vi "SysDef.Compile.vi"(8 "error in (no error)":errorcluster, 11 "Device Reference in":T1 format="%.0x") -> (0 "error out":errorcluster, 1 "Refs":T2(array[cluster]) {"VS Refs" format="%.0x"}, 2 "VS References":T3={"Name"="", "CAN"={"Interface"="", "Baud Rate"=0, "Diagnostic Protocol"=enum."GMLAN", "Transport Protocol"=enum."ISO TP - Normal Mode", "Transmit ID"=0, "Receive ID"=2, "Transmit Extension"=1, "Receive Extension"=255, "Receive UUDT ID"=0, "Enable Stream"=TRUE, "VW TP Channel ID"=1, "Fill Frame"=FALSE, "Fill Byte"=0, "Termination"=FALSE, "LIN Cluster"="", "NAD"=8, "IO Mode"=0, "Max DLC"=0, "FD Baud Rate"=2, "Security"={"Type"=enum."None", "Source DLL Path"=path "", "Target DLL Path"=path "", "Security Level"=0, "Master Key"=""}, "Timeout"=1}, "986x"={"Enable"=FALSE, "RIO Device"="", "Bitfile"=path ""}, "Reads"=[], "Frames Lookup"=variant(enum16{"GMLAN", "KWP-2000", "UDS"} enum."GMLAN"), "Writes"=[], "DPIDs"=[], "DPID Lookup"=variant(u32 0), "DTC"={"Descriptor"={"DTC Byte Length"=1, "Status Byte Length"=1, "Add Data Byte Length"=1, "Byte Order"=enum."Motorola"}, "Value.Code"=[], "Value.String"=[], "Value.J2012String"=[], "Status.Code"=[], "Status.String"=[]}, "Created DTCs"=0, "Polls"=[], "Service Channels Status Lookup"=variant, "Trigger Lookup"=variant} {"Writes"."Signals"."Byte Order" items=["Little Endian", "Big Endian"]; "Writes"."Signals"."Data Type" items=["Signed", "Unsigned", "IEEE Float"]; "CAN"."IO Mode" items=["CAN 2.0", "CAN FD", "CAN FD+BRS"]; "CAN"."Fill Byte" format="%.0x"; "CAN"."VW TP Channel ID" format="%.0x"; "CAN"."Receive UUDT ID" format="%.0x"; "CAN"."Receive Extension" format="%.0x"; "CAN"."Transmit Extension" format="%.0x"; "CAN"."Receive ID" format="%.0x"; "CAN"."Transmit ID" format="%.0x"; "Reads"."Signals"."Byte Order" items=["Little Endian", "Big Endian"]; "Reads"."Signals"."Data Type" items=["Signed", "Unsigned", "IEEE Float"]}, 3 "Device Reference out":T1 format="%.0x")   [LabVIEW 2019, in "Diagnostics Addon System Explorer.lvlib"]
uses:
  Diagnostics Addon System Explorer.lvlib
  <vilib>/NI VeriStand/Custom Device API/Custom Device Item Ref.ctl
  Shared/Types/SysDef.Compile.ctl
  Shared/Types/CAN.ctl
  Shared/Types/CAN.Interface.ctl
  Shared/Types/Protocol.ctl
  Shared/Types/Transport.ctl
  Shared/Types/Security.ctl
  Shared/Types/Security.Type.ctl
  Shared/Types/986x.ctl
  Shared/Types/Frame.Compile.ctl
  Shared/Types/Type.ctl
  Shared/Types/Signal.ctl
  Shared/Types/DPID.ctl
  Shared/Types/DPID.Rate.ctl
  Shared/Types/DTC.Settings.ctl
  Shared/Types/DTC.Descriptor.ctl
  Shared/Types/Poll.Compiled.ctl
  Types/FG.Action.ctl
  Signals.Get.vi
  Type.FG.vi
  ServiceChannels.GetRefs.vi
  SettingChannels.GetRefs.vi
  FileDependency.Create.vi
  Shared/SubVIs/Frame.Get.Size.vi
  Shared/SubVIs/LookupID.Create.vi
  Signal.FG.vi
  Frame.GetSignalRefs.vi
  Shared/SubVIs/Constants.vi
  <vilib>/NI VeriStand/Custom Device Tools/Custom Device Utility Library/NI VeriStand - Search for Item by GUID.vi
  <vilib>/NI VeriStand/Custom Device Tools/Custom Device Utility Library/NI VeriStand - Search for Item by Name.vi
  <vilib>/NI VeriStand/Custom Device API/NI VeriStand - Get Item Children.vi
  <vilib>/NI/NI VeriStand Advanced SysDef API/SysDef API/SysDef.Property.Set.vi
  <vilib>/NI/NI VeriStand Advanced SysDef API/_SubVIs/SysDef.Property.Set.U32.vi
  <vilib>/NI VeriStand/Custom Device API/NI VeriStand - Get Item Property.vi
  <vilib>/NI VeriStand/Custom Device API/Get Item Property (U32).vi
  <vilib>/NI/NI VeriStand Advanced SysDef API/_SubVIs/SysDef.Property.Set.DBL.vi
  <vilib>/NI/NI VeriStand Advanced SysDef API/_SubVIs/SysDef.Property.Set.String.vi
  <vilib>/NI VeriStand/Custom Device API/Get Item Property (Double).vi
  <vilib>/NI VeriStand/Custom Device API/Get Item Property (String).vi
  <vilib>/NI VeriStand/Custom Device API/NI VeriStand - Get Item Description.vi
  <vilib>/NI VeriStand/Custom Device API/NI VeriStand - Get Custom Device Channel Data.vi
  <vilib>/NI VeriStand/Custom Device Tools/Custom Device Utility Library/NI VeriStand - Search for All Items by GUID.vi
  <vilib>/NI/NI VeriStand Advanced SysDef API/_SubVIs/SysDef.Property.Set.I32.vi
  <vilib>/NI/NI VeriStand Advanced SysDef API/_SubVIs/SysDef.Property.Set.DBL.Array.vi
  <vilib>/NI/NI VeriStand Advanced SysDef API/_SubVIs/SysDef.Property.Set.String.Array.vi
  <vilib>/NI VeriStand/Custom Device API/Get Item Property (I32).vi
  <vilib>/NI VeriStand/Custom Device API/Get Item Property (Double Array).vi
  <vilib>/NI VeriStand/Custom Device API/Get Item Property (String Array).vi
  <vilib>/NI VeriStand/Custom Device API/Get Item Property (Variant).vi
  <vilib>/NI VeriStand/Custom Device API/Get Item Property (Boolean).vi
  FileDependency.Get.Target Path.vi
  <vilib>/NI/NI VeriStand Advanced SysDef API/_SubVIs/SysDef.Property.Set.Variant.vi
  <vilib>/NI/NI VeriStand Advanced SysDef API/_SubVIs/SysDef.Property.Set.Boolean.vi
  <vilib>/Utility/MD5Checksum.llb/MD5Checksum File.vi
  <vilib>/NI/NI VeriStand Advanced SysDef API/_SubVIs/SysDef.Property.Set.DependentFile.vi
  <vilib>/NI/NI VeriStand Advanced SysDef API/SysDef API/SysDef.Property.Remove.vi
  <vilib>/NI/NI VeriStand Advanced SysDef API/_SubVIs/SysDef.Property.Set.U32.Array.vi
  <vilib>/NI VeriStand/Custom Device API/Get Item Property (U32 Array).vi
  <vilib>/NI VeriStand/Custom Device Tools/Custom Device Utility Library/Custom Device Utility Library.lvlib
  Shared/Diagnostics Addon Shared.lvlib
  <vilib>/NI VeriStand/Custom Device API/Custom Device API.lvlib
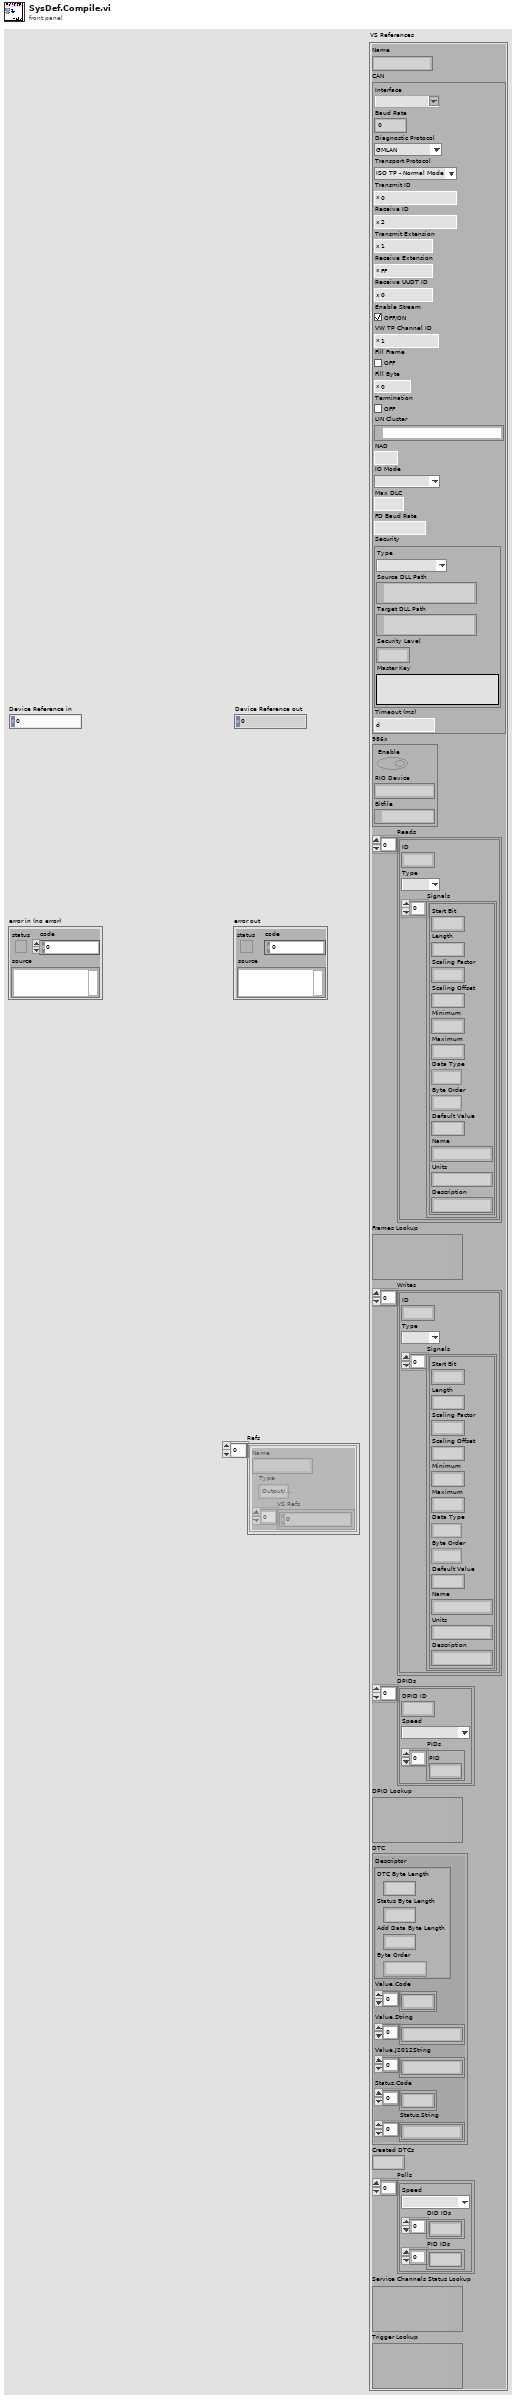
[diagram p1: front panel]
types:
  T1 = typedef "Custom Device API.lvlib/Custom Device Item Ref.ctl" = u64
  T2 = cluster{"Name":string, "Type":enum16{"Output/Write", "Input/Read", "Input/ReadWrite"}, "VS Refs":T1[]}[]
  T3 = typedef "Diagnostics Addon Shared.lvlib/SysDef.Compile.ctl" = cluster{"Name":string, "CAN":T4, "986x":T10, "Reads":T11[], "Frames Lookup":variant, "Writes":T11[], "DPIDs":T14[], "DPID Lookup":variant, "DTC":T16, "Created DTCs":u32, "Polls":T18[], "Service Channels Status Lookup":variant, "Trigger Lookup":variant}
  T4 = typedef "Diagnostics Addon Shared.lvlib/CAN.ctl" = cluster{"Interface":T5, "Baud Rate":u64, "Diagnostic Protocol":T6, "Transport Protocol":T7, "Transmit ID":u32, "Receive ID":u32, "Transmit Extension":u8, "Receive Extension":u8, "Receive UUDT ID":u32, "Enable Stream":bool, "VW TP Channel ID":u32, "Fill Frame":bool, "Fill Byte":u8, "Termination":bool, "LIN Cluster":refnum<k21>, "NAD":u8, "IO Mode":u32, "Max DLC":u16, "FD Baud Rate":u64, "Security":T8, "Timeout":u32}
  T5 = typedef "Diagnostics Addon Shared.lvlib/CAN.Interface.ctl" = string
  T6 = typedef "Diagnostics Addon Shared.lvlib/Protocol.ctl" = enum16{"GMLAN", "KWP-2000", "UDS", "User-Defined"}
  T7 = typedef "Diagnostics Addon Shared.lvlib/Transport.ctl" = enum16{"ISO TP - Normal Mode", "ISO TP - Mixed Mode", "VW TP 2.0", "Diagnostics on IP", "ISO TP LIN"}
  T8 = typedef "Diagnostics Addon Shared.lvlib/Security.ctl" = cluster{"Type":T9, "Source DLL Path":path, "Target DLL Path":path, "Security Level":u8, "Master Key":string}
  T9 = typedef "Diagnostics Addon Shared.lvlib/Security.Type.ctl" = enum16{"None", "DLL", "MasterKey"}
  T10 = typedef "Diagnostics Addon Shared.lvlib/986x.ctl" = cluster{"Enable":bool, "RIO Device":string, "Bitfile":path}
  T11 = typedef "Diagnostics Addon Shared.lvlib/Frame.Compile.ctl" = cluster{"ID":u32, "Type":T12, "Signals":T13[]}
  T12 = typedef "Diagnostics Addon Shared.lvlib/Type.ctl" = enum16{"DID", "CDID", "PID", "CPID", "Read Memory", "Write Memory", "IO Control", "Routine Start", "Routine Request", "Routine Stop", "User Defined", "DTC Control", "Clear DTCs", "Read DTCs", "Start DTCs", "DTC Change Count", "Tester Present", "Unlock ECU", "Reset ECU", "Diag Session Control", "Communication Control", "Configure DPIDs", "Start DPIDs", "Stop DPIDs"}
  T13 = typedef "Diagnostics Addon Shared.lvlib/Signal.ctl" = cluster{"Start Bit":u32, "Length":u32, "Scaling Factor":dbl, "Scaling Offset":dbl, "Minimum":dbl, "Maximum":dbl, "Data Type":u32, "Byte Order":u32, "Default Value":dbl, "Name":string, "Units":string, "Description":string}
  T14 = typedef "Diagnostics Addon Shared.lvlib/DPID.ctl" = cluster{"DPID ID":u8, "Speed":T15, "PIDs":u16[]}
  T15 = typedef "Diagnostics Addon Shared.lvlib/DPID.Rate.ctl" = enum16{"Slow", "Medium", "Fast"}
  T16 = typedef "Diagnostics Addon Shared.lvlib/DTC.Settings.ctl" = cluster{"Descriptor":T17, "Value.Code":dbl[], "Value.String":string[], "Value.J2012String":string[], "Status.Code":dbl[], "Status.String":string[]}
  T17 = typedef "Diagnostics Addon Shared.lvlib/DTC.Descriptor.ctl" = cluster{"DTC Byte Length":i32, "Status Byte Length":i32, "Add Data Byte Length":i32, "Byte Order":enum16{"Motorola", "Intel"}}
  T18 = typedef "Diagnostics Addon Shared.lvlib/Poll.Compiled.ctl" = cluster{"Speed":T15, "DID IDs":u32[], "PID IDs":u32[]}
  T19 = enum16{"Output/Write", "Input/Read", "Input/ReadWrite"}
  T20 = cluster{"Name":string, "Type":enum16{"Output/Write", "Input/Read", "Input/ReadWrite"}, "VS Refs":T1[]}
  T21 = typedef "Diagnostics Addon System Explorer.lvlib/FG.Action.ctl" = enum16{"Get", "Set"}
  T22 = typedef "Diagnostics Addon System Explorer.lvlib/Service.Export.ctl" = cluster{"Signal.Cmd.Refs":T23[], "Signal.Cmd.Info":T11[], "Signal.Resp.Refs":T23[], "Signal.Resp.Info":T11[], "Trigger.Refs":T23[], "Status.Refs":T23[], "Settings.Refs":T23[]}
  T23 = typedef "Diagnostics Addon System Explorer.lvlib/Frame.Ref.ctl" = cluster{"Type":T12, "ID":u32, "Signal Refs":T1[]}
  T24 = typedef "Diagnostics Addon System Explorer.lvlib/Poll.LinkedNode.ctl" = cluster{"Node ID":u64}
  T25 = typedef "Custom Device API.lvlib/Custom Device Item Info.ctl" = cluster{"Name":string, "Is Channel":bool, "GUID":string, "Is Waveform":bool}
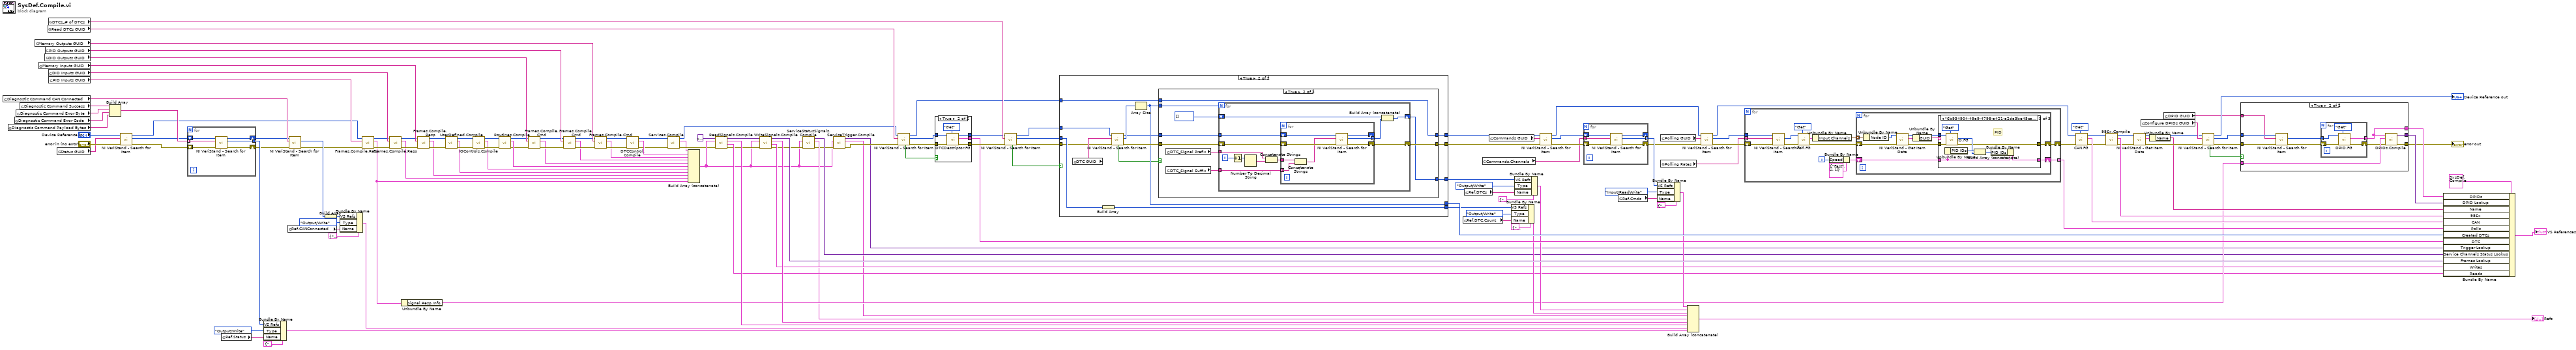
[diagram p0: block diagram]
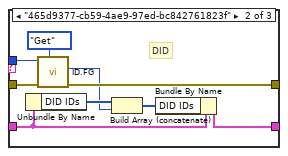
[diagram p6: hidden frame]
diagram:
  n1 = global read "Constants.vi" "Diagnostic Command CAN Connected"() -> (w55:string)
  n2 = global read "Constants.vi" "Diagnostic Command Payload Bytes"() -> (w99:string)
  n3 = global read "Constants.vi" "Diagnostic Command Error Code"() -> (w98:string)
  n4 = global read "Constants.vi" "Diagnostic Command Error Byte"() -> (w100:string)
  n5 = global read "Constants.vi" "Diagnostic Command Success"() -> (w101:string)
  n6 = global read "Constants.vi" "Memory Outputs GUID"() -> (w118:string)
  n7 = global read "Constants.vi" "Memory Inputs GUID"() -> (w117:string)
  n8 = global read "Constants.vi" "DID Outputs GUID"() -> (w93:string)
  n9 = global read "Constants.vi" "PID Outputs GUID"() -> (w145:string)
  n10 = global read "Constants.vi" "Read DTCs GUID"() -> (w149:string)
  n11 = global read "Constants.vi" "DTCs_# of DTCs"() -> (w148:string)
  n12 = global read "Constants.vi" "DID Inputs GUID"() -> (w146:string)
  n13 = global read "Constants.vi" "PID Inputs GUID"() -> (w144:string)
  n14 = global read "Constants.vi" "Status GUID"() -> (w41:string)
  n15 = Build Array(w101, w100, w98, w99) -> (w97:string[])
  n16 = call-poly <vilib>:"NI VeriStand - Search for Item.vi"("error in"="error in (no error)", "Item GUID"=w41, "Section Ref in"="Device Reference in") -> ("error out"=w43:errorcluster, "Item Ref"=w45:T1, "Section Ref out"=w42:T1)  [unwired: 5 in, 1 out]
  n17 = for {
    tunnel: w97 -> [w153] mode=indexing
    tunnel: [w152] -> w75 mode=indexing
    shift-right: [w151] -> w50
    shift-left: w43 -> [w155]
    shift-right: [w150] -> w48
    shift-left: w45 -> [w154]
    n18 = call-poly <vilib>:"NI VeriStand - Search for Item.vi"("error in"=w155, "Item Name"=w153, "Section Ref in"=w154) -> ("error out"=w151:errorcluster, "Item Ref"=w152:T1, "Section Ref out"=w150:T1)  [unwired: 5 in, 1 out]
  }
  n19 = global read "Constants.vi" "Ref.Status"() -> (w83:string)
  n20 = Bundle By Name(cluster=T20 {"Name"="", "Type"=enum."Output/Write", "VS Refs"=[]} ("Group"), "VS Refs"=w75, "Type"=T19."Output/Write", "Name"=w83) -> (w71:T20)
  n21 = global read "Constants.vi" "Ref.CANConnected"() -> (w54:string)
  n22 = call-poly <vilib>:"NI VeriStand - Search for Item.vi"("error in"=w50, "Item Name"=w55, "Section Ref in"=w48) -> ("error out"=w49:errorcluster, "Item Ref"=w52:T1)  [unwired: 5 in, 2 out]
  n23 = Build Array(w52) -> (w51:T1[])
  n24 = Bundle By Name(cluster=T20 {"Name"="", "Type"=enum."Output/Write", "VS Refs"=[]} ("Group"), "VS Refs"=w51, "Type"=T19."Output/Write", "Name"=w54) -> (w40:T20)
  n25 = call "Frames.Compile.Resp.vi"("error in (no error)"=w49, "GUID"=w144, "Section Ref in"=w42) -> ("error out"=w111:errorcluster, "Settings"=w26:T22, "Section Ref out"=w116:T1)  [unwired: 6 in]
  n26 = call "Frames.Compile.Resp.vi"("error in (no error)"=w111, "GUID"=w146, "Section Ref in"=w116) -> ("error out"=w112:errorcluster, "Settings"=w27:T22, "Section Ref out"=w115:T1)  [unwired: 6 in]
  n27 = Unbundle By Name(w26) -> ("Signal.Resp.Info"=w30:T11[])
  n28 = call "Frames.Compile.Resp.vi"("error in (no error)"=w112, "GUID"=w117, "Section Ref in"=w115) -> ("error out"=w91:errorcluster, "Settings"=w28:T22, "Section Ref out"=w92:T1)  [unwired: 6 in]
  n29 = call "UserDefined.Compile.vi"("error in (no error)"=w91, "Section Ref in"=w92) -> ("error out"=w90:errorcluster, "Settings"=w24:T22, "Section Ref out"=w89:T1)  [unwired: 7 in]
  n30 = call "IOControls.Compile.vi"("error in (no error)"=w90, "Section Ref in"=w89) -> ("error out"=w113:errorcluster, "Settings"=w23:T22, "Section Ref out"=w114:T1)  [unwired: 7 in]
  n31 = call "Routines.Compile.vi"("error in (no error)"=w113, "Section Ref in"=w114) -> ("error out"=w17:errorcluster, "Settings"=w22:T22, "Section Ref out"=w16:T1)  [unwired: 7 in]
  n32 = call "Frames.Compile.Cmd.vi"("error in (no error)"=w17, "GUID"=w93, "Section Ref in"=w16) -> ("error out"=w94:errorcluster, "Settings"=w18:T22, "Section Ref out"=w95:T1)  [unwired: 6 in]
  n33 = call "Frames.Compile.Cmd.vi"("error in (no error)"=w94, "GUID"=w145, "Section Ref in"=w95) -> ("error out"=w105:errorcluster, "Settings"=w19:T22, "Section Ref out"=w108:T1)  [unwired: 6 in]
  n34 = call "Frames.Compile.Cmd.vi"("error in (no error)"=w105, "GUID"=w118, "Section Ref in"=w108) -> ("error out"=w106:errorcluster, "Settings"=w20:T22, "Section Ref out"=w107:T1)  [unwired: 6 in]
  n35 = call "DTCControl.Compile.vi"("error in (no error)"=w106, "Section Ref in"=w107) -> ("error out"=w5:errorcluster, "Settings"=w21:T22, "Section Ref out"=w3:T1)  [unwired: 7 in]
  n36 = call "Services.Compile.vi"("error in (no error)"=w5, "Section Ref in"=w3) -> ("error out"=w4:errorcluster, "Settings"=w1:T22[], "Section Ref out"=w2:T1)  [unwired: 7 in]
  n37 = Build Array (concatenate)(w1, w21, w20, w19, w18, w22, w23, w24, w28, w27, w26) -> (w9:T22[])
  n38 = call "ReadSignals.Compile.vi"("error in (no error)"=w4, "Settings"=w9, "Lookups in"=variant) -> ("error out"=w15:errorcluster, "Signal Info"=w29:T11[], "Refs"=w72:T20, "Lookups"=w80:variant)  [unwired: 5 in]
  n39 = call "WriteSignals.Compile.vi"("error in (no error)"=w15, "Settings"=w9, "Lookup In"=w80) -> ("error out"=w14:errorcluster, "Signal Info"=w25:T11[], "Refs"=w73:T20, "Lookup"=w79:variant)  [unwired: 5 in]
  n40 = call "ServiceStatusSignals.Compile.vi"("error in (no error)"=w14, "Settings"=w9) -> ("error out"=w11:errorcluster, "Refs"=w13:T20, "Status Lookup"=w12:variant)  [unwired: 7 in]
  n41 = call "ServiceTrigger.Compile.vi"("error in (no error)"=w11, "Settings"=w9) -> ("error out"=w10:errorcluster, "Refs"=w8:T2, "Trigger Lookup"=w7:variant)  [unwired: 7 in]
  n42 = call-poly <vilib>:"NI VeriStand - Search for Item.vi"("error in"=w10, "Item GUID"=w149, "Section Ref in"=w2) -> ("error out"=w136:errorcluster, "Item Ref"=w134:T1, "Section Ref out"=w96:T1, "Found"=w86:bool)  [unwired: 5 in]
  n43 = case shown="True" w86 {
    tunnel: w136 -> [w157 w162]
    tunnel: [w157 w161] -> w135
    tunnel: w134 -> [w156 w160]
    tunnel: [w156 w159] -> w133
    tunnel: [_ w158] -> w132
    frame False {
    }
    frame True {
      n44 = call "DTCDescriptor.FG.vi"("Action"=FG.Action."Get", "error in (no error)"=w162, "Device Item Ref in"=w160) -> ("error out"=w161:errorcluster, "DTC descriptor"=w158:T16, "Device Item Ref out"=w159:T1)  [unwired: 6 in]
    }
  }
  n45 = call-poly <vilib>:"NI VeriStand - Search for Item.vi"("error in"=w135, "Item Name"=w148, "Section Ref in"=w133) -> ("error out"=w142:errorcluster, "Item Ref"=w143:T1, "Section Ref out"=w88:T1, "Found"=w85:bool)  [unwired: 5 in]
  n46 = case shown="True" w85 {
    tunnel: w143 -> [_ w169]
    tunnel: w142 -> [w164 w168]
    tunnel: [_ w179] -> w65
    tunnel: [w164 w178] -> w110
    tunnel: [w165 w177] -> w109
    tunnel: w96 -> [w165 w167]
    tunnel: w88 -> [_ w174]
    tunnel: [_ w171] -> w87
    tunnel: [_ w166] -> w61
    frame False {
    }
    frame True {
      n47 = global read "Constants.vi" "DTC GUID"() -> (w172:string)
      n48 = Build Array(w169) -> (w166:T1[])
      n49 = call-poly <vilib>:"NI VeriStand - Search for Item.vi"("error in"=w168, "Item GUID"=w172, "Section Ref in"=w174) -> ("error out"=w176:errorcluster, "Item Refs"=w175:T1[], "Section Ref out"=w173:T1, "Found"=w170:bool)  [unwired: 5 in]
      n50 = Array Size(array=w175) -> (size(s)=w171:i32)
      n51 = case shown="True" w170 {
        tunnel: [_ w182] -> w179
        tunnel: [w180 w184] -> w178
        tunnel: [w181 w183] -> w177
        tunnel: w167 -> [w181 w183]
        tunnel: w176 -> [w180 w187]
        tunnel: w173 -> [_ w186]
        tunnel: w171 -> [_ w185]
        frame False {
        }
        frame True {
          n52 = global read "Constants.vi" "DTC_Signal Prefix"() -> (w190:string)
          n53 = global read "Constants.vi" "DTC_Signal Suffix"() -> (w189:string[])
          n54 = for {
            N: w185 -> [_]
            tunnel: w186 -> [w202]
            shift-right: [w200] -> w184
            shift-left: w187 -> [w201]
            tunnel: w189 -> [w195]
            tunnel: w190 -> [w194]
            shift-right: [w191] -> w182
            shift-left: T1[] [] -> [w193]
            i -> [w197]
            n55 = Increment(x=w197) -> (x+1=w199:i32)
            n56 = Number To Decimal String(number=w199) -> (decimal integer string=w198:string)  [unwired: 1 in]
            n57 = Concatenate Strings(w194, w198) -> (w196:string)
            n58 = for {
              shift-right: [w209] -> _
              shift-left: w202 -> [w210]
              shift-right: [w207] -> w200
              shift-left: w201 -> [w208]
              tunnel: w195 -> [w206] mode=indexing
              tunnel: w196 -> [w205]
              tunnel: [w203] -> w192 mode=indexing
              n59 = Concatenate Strings(w205, w206) -> (w204:string)
              n60 = call-poly <vilib>:"NI VeriStand - Search for Item.vi"("error in"=w208, "Item Name"=w204, "Section Ref in"=w210) -> ("error out"=w207:errorcluster, "Item Ref"=w203:T1, "Section Ref out"=w209:T1)  [unwired: 5 in, 1 out]
            }
            n61 = Build Array (concatenate)(w193, w192) -> (w191:T1[])
          }
        }
      }
    }
  }
  n62 = global read "Constants.vi" "Ref.DTC.Count"() -> (w63:string)
  n63 = global read "Constants.vi" "Ref.DTCs"() -> (w68:string)
  n64 = global read "Constants.vi" "Commands.Channels"() -> (w57:string[])
  n65 = global read "Constants.vi" "Commands GUID"() -> (w147:string)
  n66 = Bundle By Name(cluster=T20 {"Name"="", "Type"=enum."Output/Write", "VS Refs"=[]} ("Group"), "VS Refs"=w61, "Type"=T19."Output/Write", "Name"=w63) -> (w60:T20)
  n67 = Bundle By Name(cluster=T20 {"Name"="", "Type"=enum."Output/Write", "VS Refs"=[]} ("Group"), "VS Refs"=w65, "Type"=T19."Output/Write", "Name"=w68) -> (w66:T20)
  n68 = call-poly <vilib>:"NI VeriStand - Search for Item.vi"("error in"=w110, "Item GUID"=w147, "Section Ref in"=w109) -> ("error out"=w59:errorcluster, "Item Ref"=w58:T1, "Section Ref out"=w37:T1)  [unwired: 5 in, 1 out]
  n69 = for {
    shift-right: [w214] -> w38
    shift-left: w59 -> [w216]
    tunnel: w57 -> [w213] mode=indexing
    tunnel: [w212] -> w56 mode=indexing
    shift-right: [w211] -> _
    shift-left: w58 -> [w215]
    n70 = call-poly <vilib>:"NI VeriStand - Search for Item.vi"("error in"=w216, "Item Name"=w213, "Section Ref in"=w215) -> ("error out"=w214:errorcluster, "Item Ref"=w212:T1, "Section Ref out"=w211:T1)  [unwired: 5 in, 1 out]
  }
  n71 = global read "Constants.vi" "Ref.Cmds"() -> (w77:string)
  n72 = Bundle By Name(cluster=T20 {"Name"="", "Type"=enum."Output/Write", "VS Refs"=[]} ("Group"), "VS Refs"=w56, "Type"=T19."Input/ReadWrite", "Name"=w77) -> (w74:T20)
  n73 = global read "Constants.vi" "Polling GUID"() -> (w39:string)
  n74 = global read "Constants.vi" "Polling Rates"() -> (w33:string[])
  n75 = Build Array (concatenate)(w74, w66, w60, w8, w13, w73, w72, w40, w71) -> (→"Refs":T2)
  n76 = call-poly <vilib>:"NI VeriStand - Search for Item.vi"("error in"=w38, "Item GUID"=w39, "Section Ref in"=w37) -> ("error out"=w35:errorcluster, "Item Ref"=w34:T1, "Section Ref out"=w36:T1)  [unwired: 5 in, 1 out]
  n77 = for {
    tunnel: w34 -> [w229]
    shift-right: [w217] -> w32
    shift-left: w35 -> [w230]
    tunnel: w33 -> [w228] mode=indexing
    tunnel: [w218] -> w31 mode=indexing
    i -> [w224]
    n78 = call-poly <vilib>:"NI VeriStand - Search for Item.vi"("error in"=w230, "Item Name"=w228, "Section Ref in"=w229) -> ("error out"=w227:errorcluster, "Item Ref"=w226:T1)  [unwired: 5 in, 2 out]
    n79 = call "Poll.FG.vi"("Action"=FG.Action."Get", "error in"=w227, "Parent Ref"=w226) -> ("error out"=w220:errorcluster, "Selected Channels out"=w222:cluster{"Input Channels":T24[]})  [unwired: 6 in, 1 out]
    n80 = Unbundle By Name(w222) -> ("Input Channels"=w221:T24[])
    n81 = Bundle By Name(cluster=T18 {"Speed"=enum."Fast", "DID IDs"=[], "PID IDs"=[]}, "Speed"=w224) -> (w219:T18)
    n82 = for {
      tunnel: w221 -> [w240] mode=indexing
      shift-right: [w233] -> w217
      shift-left: w220 -> [w238]
      shift-right: [w232] -> w218
      shift-left: w219 -> [w234]
      n83 = Unbundle By Name(w240) -> ("Node ID"=w237:u64)
      n84 = call <vilib>:"NI VeriStand - Get Item Data.vi"("error in (no error)"=w238, "Item Ref in"=w237) -> ("error out"=w235:errorcluster, "Item Info"=w239:T25, "Item Ref out"=w231:T1)  [unwired: 6 in, 1 out]
      n85 = Unbundle By Name(w239) -> ("GUID"=w236:string)
      n86 = case shown="\"6b934904-49a9-4798-a421-a2da3be45ca1\"" w236 {
        tunnel: w235 -> [w242 w250 w259]
        tunnel: w234 -> [w241 w248 w256]
        tunnel: [w242 w249 w253] -> w233
        tunnel: [w241 w243 w252] -> w232
        tunnel: w231 -> [_ w245 w255]
        frame Default {
        }
        frame "465d9377-cb59-4ae9-97ed-bc842761823f" {
          # "DID"
          n87 = Unbundle By Name(w248) -> ("DID IDs"=w247:u32[])
          n88 = call "ID.FG.vi"("Action"=FG.Action."Get", "error in (no error)"=w250, "Device Item Ref in"=w245) -> ("error out"=w249:errorcluster, "ID"=w246:u32)  [unwired: 6 in, 1 out]
          n89 = Build Array (concatenate)(w247, w246) -> (w244:u32[])
          n90 = Bundle By Name(cluster=w248, "DID IDs"=w244) -> (w243:T18)
        }
        frame "6b934904-49a9-4798-a421-a2da3be45ca1" {
          # "PID"
          n91 = Unbundle By Name(w256) -> ("PID IDs"=w258:u32[])
          n92 = call "ID.FG.vi"("Action"=FG.Action."Get", "error in (no error)"=w259, "Device Item Ref in"=w255) -> ("error out"=w253:errorcluster, "ID"=w254:u32)  [unwired: 6 in, 1 out]
          n93 = Build Array (concatenate)(w258, w254) -> (w257:u32[])
          n94 = Bundle By Name(cluster=w256, "PID IDs"=w257) -> (w252:T18)
        }
      }
    }
  }
  n95 = call "CAN.FG.vi"("Action"=FG.Action."Get", "error in (no error)"=w32, "Device Item Ref in"=w36) -> ("error out"=w129:errorcluster, "Diagnostics Basic Configuration"=w130:T4, "Device Item Ref out"=w128:T1)  [unwired: 6 in]
  n96 = call "986x.Compile.vi"("error in (no error)"=w129, "Item Ref in"=w128) -> ("error out"=w124:errorcluster, "986x Support"=w127:T10, "Item Ref out"=w122:T1)  [unwired: 7 in]
  n97 = call <vilib>:"NI VeriStand - Get Item Data.vi"("error in (no error)"=w124, "Item Ref in"=w122) -> ("error out"=w123:errorcluster, "Item Info"=w125:T25, "Item Ref out"=w121:T1)  [unwired: 6 in, 1 out]
  n98 = global read "Constants.vi" "Configure DPIDs GUID"() -> (w140:string)
  n99 = Unbundle By Name(w125) -> ("Name"=w120:string)
  n100 = global read "Constants.vi" "DPID GUID"() -> (w6:string)
  n101 = call-poly <vilib>:"NI VeriStand - Search for Item.vi"("error in"=w123, "Item GUID"=w140, "Section Ref in"=w121) -> ("error out"=w141:errorcluster, "Item Ref"=w139:T1, "Section Ref out"=→"Device Reference out":T1, "Found"=w137:bool)  [unwired: 5 in]
  n102 = case shown="True" w137 {
    tunnel: w141 -> [w261 w266]
    tunnel: w139 -> [_ w265]
    tunnel: [w261 w269] -> w103
    tunnel: [_ w267] -> w131
    tunnel: w30 -> [_ w271]
    tunnel: [_ w268] -> w119
    tunnel: w6 -> [_ w264]
    frame False {
    }
    frame True {
      n103 = call-poly <vilib>:"NI VeriStand - Search for Item.vi"("error in"=w266, "Item GUID"=w264, "Section Ref in"=w265) -> ("error out"=w263:errorcluster, "Item Refs"=w262:T1[])  [unwired: 5 in, 2 out]
      n104 = for {
        tunnel: w262 -> [w275] mode=indexing
        tunnel: [w274] -> w267 mode=indexing
        shift-right: [w273] -> w270
        shift-left: w263 -> [w276]
        n105 = call "DPID.FG.vi"("Action"=FG.Action."Get", "error in (no error)"=w276, "Device Item Ref in"=w275) -> ("error out"=w273:errorcluster, "DPID"=w274:T14)  [unwired: 6 in, 1 out]
      }
      n106 = call "DPIDs.Compile.vi"("error in (no error)"=w270, "PIDs"=w271, "DPIDs"=w267) -> ("error out"=w269:errorcluster, "Lookup Table"=w268:variant)  [unwired: 7 in]
    }
  }
  "error out" <- w103
  n107 = Bundle By Name(cluster=T3 {"Name"="", "CAN"={"Interface"="", "Baud Rate"=0, "Diagnostic Protocol"=enum."GMLAN", "Transport Protocol"=enum."ISO TP - Normal Mode", "Transmit ID"=0, "Receive ID"=2, "Transmit Extension"=1, "Receive Extension"=255, "Receive UUDT ID"=0, "Enable Stream"=TRUE, "VW TP Channel ID"=1, "Fill Frame"=FALSE, "Fill Byte"=0, "Termination"=FALSE, "LIN Cluster"="", "NAD"=8, "IO Mode"=0, "Max DLC"=0, "FD Baud Rate"=2, "Security"={"Type"=enum."None", "Source DLL Path"=path "", "Target DLL Path"=path "", "Security Level"=0, "Master Key"=""}, "Timeout"=1}, "986x"={"Enable"=FALSE, "RIO Device"="", "Bitfile"=path ""}, "Reads"=[], "Frames Lookup"=variant(enum16{"GMLAN", "KWP-2000", "UDS"} enum."GMLAN"), "Writes"=[], "DPIDs"=[], "DPID Lookup"=variant(u32 0), "DTC"={"Descriptor"={"DTC Byte Length"=1, "Status Byte Length"=1, "Add Data Byte Length"=1, "Byte Order"=enum."Motorola"}, "Value.Code"=[], "Value.String"=[], "Value.J2012String"=[], "Status.Code"=[], "Status.String"=[]}, "Created DTCs"=0, "Polls"=[], "Service Channels Status Lookup"=variant, "Trigger Lookup"=variant} ("VS References"), "DPIDs"=w131, "DPID Lookup"=w119, "Name"=w120, "986x"=w127, "CAN"=w130, "Polls"=w31, "Created DTCs"=w87, "DTC"=w132, "Trigger Lookup"=w7, "Service Channels Status Lookup"=w12, "Frames Lookup"=w79, "Writes"=w25, "Reads"=w29) -> (→"VS References":T3)
